vi "zatezovaci_charakteristika.vi"() -> ()   [LabVIEW 2024]
uses:
  <vilib>/Analysis/baseanly.llb/Mean (DBL).vi
  EFmeter.lvlib
  <vilib>/Analysis/NI_AALBase.lvlib
  BK Precision 8500B Series/BK Precision 8500B Series.lvlib
  <instrlib>/Zatez Kopper/Zatez Kopper.lvlib
panel:
  in  "LOAD":refnum<visa-resource-name>
  in  "Clear":bool
  in  "Typ zateze":u16(ring) items=["Manualni", "BK 8542B", "KOPPER-zatez"]
  in  "Ulozit data":bool caption="Uložit data"
  in  "file path (use dialog)":path
  in  "Vzorku na krokù":u16 max=100 step=1
  in  "Prumerovani":bool
  in  "Start [A]":dbl
  in  "Velikost kroku [A]":dbl
  in  "EFmeter":refnum<visa-resource-name>
  out "Aktualni zatez":dbl=2.5
  out "R_out":dbl
  in  "Pocet kroku":i32
  out "Zatezovaci charakteristika":cluster{"X":dbl[], "Y":dbl[]}[](graph)
  in  "stop":bool
  in  "Start":bool
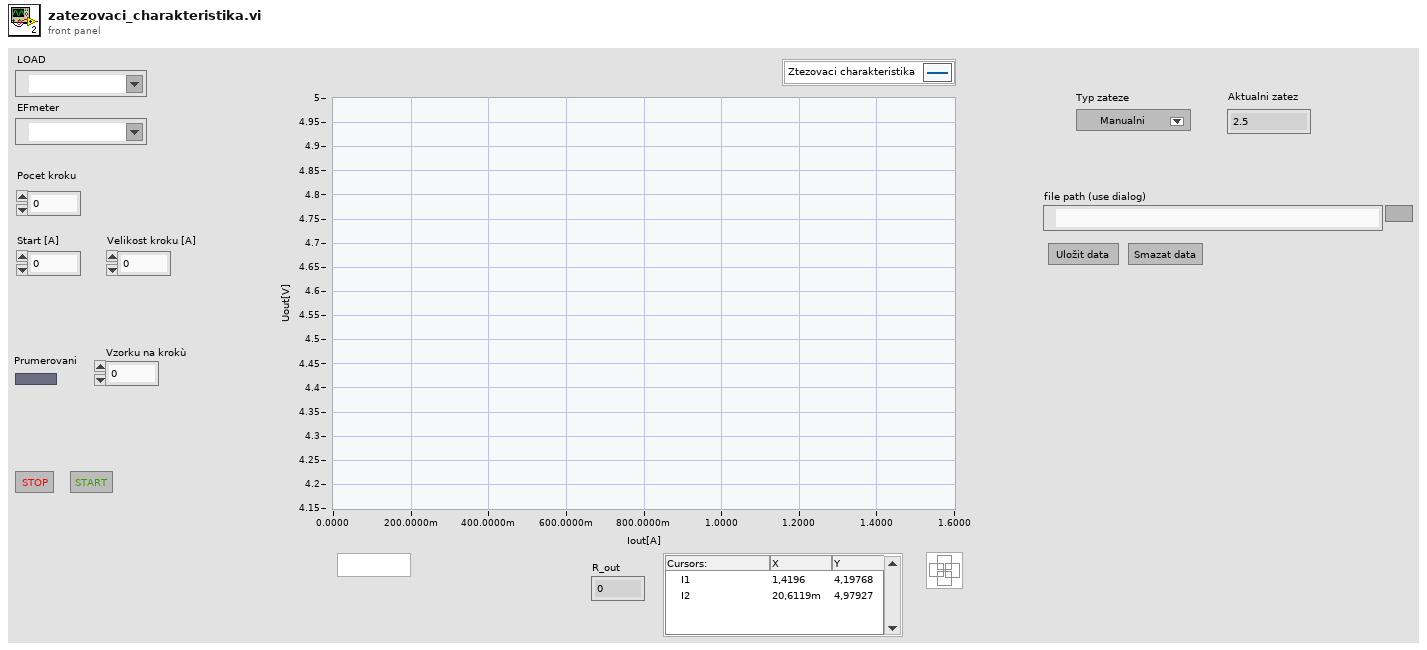
[diagram p1: front panel]
types:
  T1 = enum16{"init", "wait", "graph", "meas", "change_load", "init_measurment", "save", "clear"}
  T2 = typedef "LVCursorListTypeDef.ctl" = cluster{"Name":string, "Color":u32, "Style":u8, "Point Style":u8, "Name Visible":bool, "Allow Drag":bool, "Cursor Mode":u32, "Plot":i32, "Index":i32, "Position":cluster{"X":dbl, "Y":dbl}, "X Scale":u32, "Y Scale":u32, "Watch Plots":i32[], "Watch All Plots":bool, "Plot Area":i32, "Label Offset":cluster{"X":dbl, "Y":dbl}}[]
  T3 = cluster{"Name":string, "Color":u32, "Style":u8, "Point Style":u8, "Name Visible":bool, "Allow Drag":bool, "Cursor Mode":u32, "Plot":i32, "Index":i32, "Position":cluster{"X":dbl, "Y":dbl}, "X Scale":u32, "Y Scale":u32, "Watch Plots":i32[], "Watch All Plots":bool, "Plot Area":i32, "Label Offset":cluster{"X":dbl, "Y":dbl}}
  T4 = enum16{"open", "replace", "create", "open or create", "replace or create", "replace or create with confirmation"}
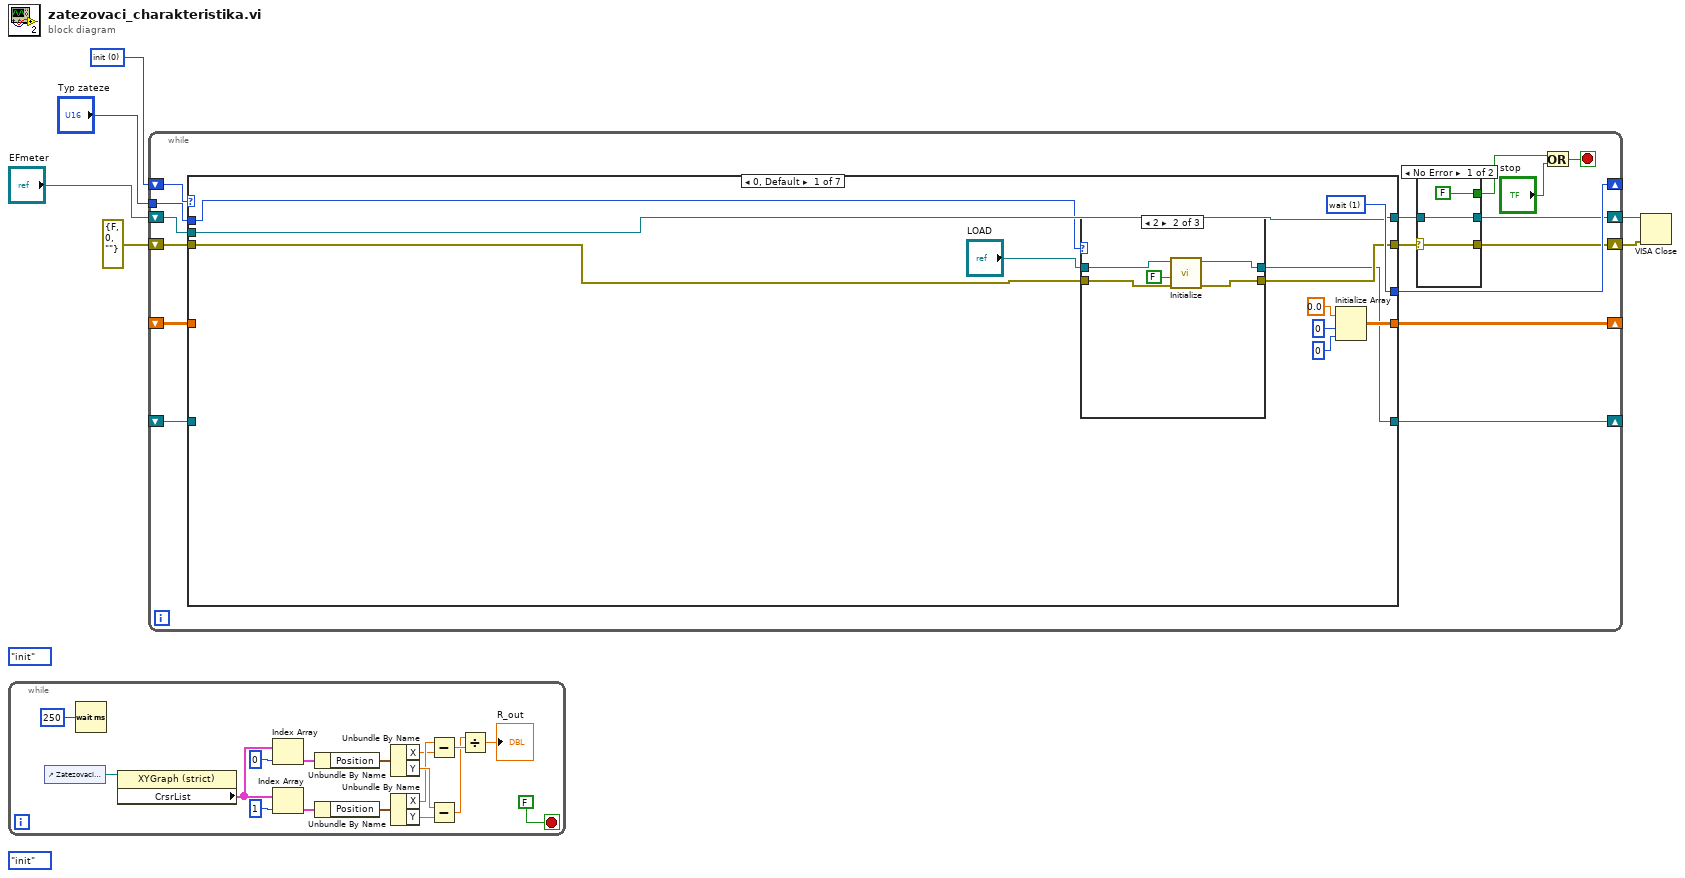
[diagram p0: block diagram]
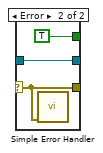
[diagram p2: hidden frame]
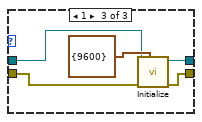
[diagram p4: hidden frame]
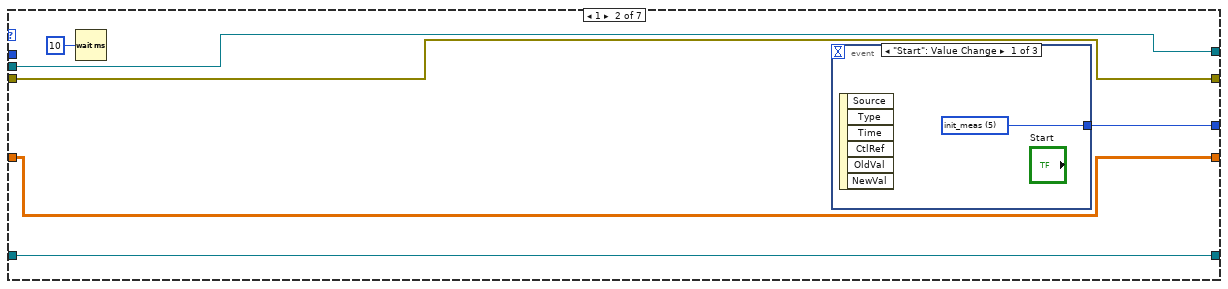
[diagram p5: hidden frame]
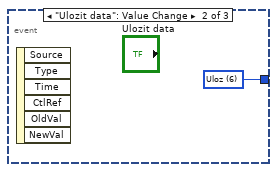
[diagram p6: hidden frame]
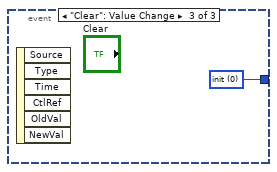
[diagram p7: hidden frame]
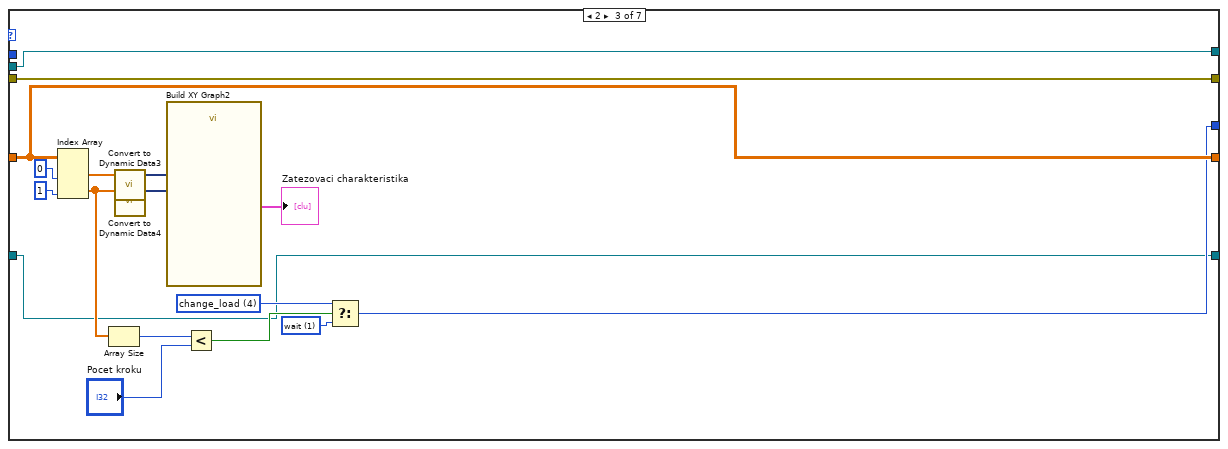
[diagram p8: hidden frame]
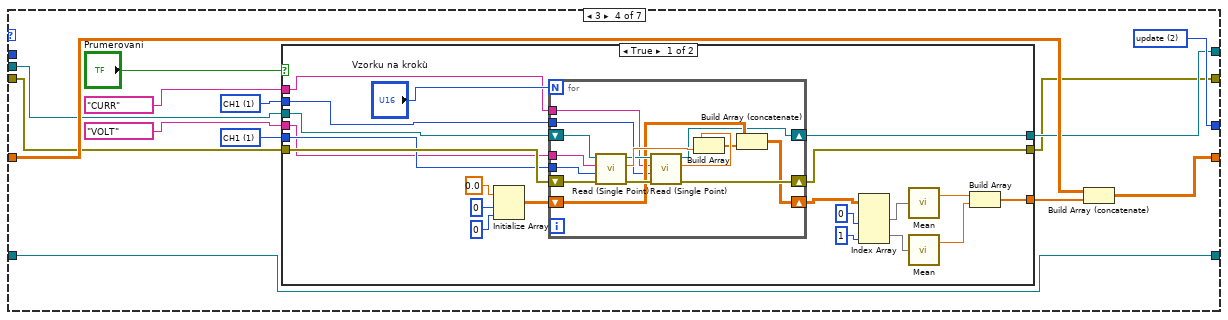
[diagram p9: hidden frame]
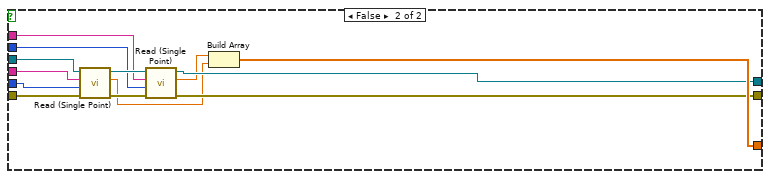
[diagram p10: hidden frame]
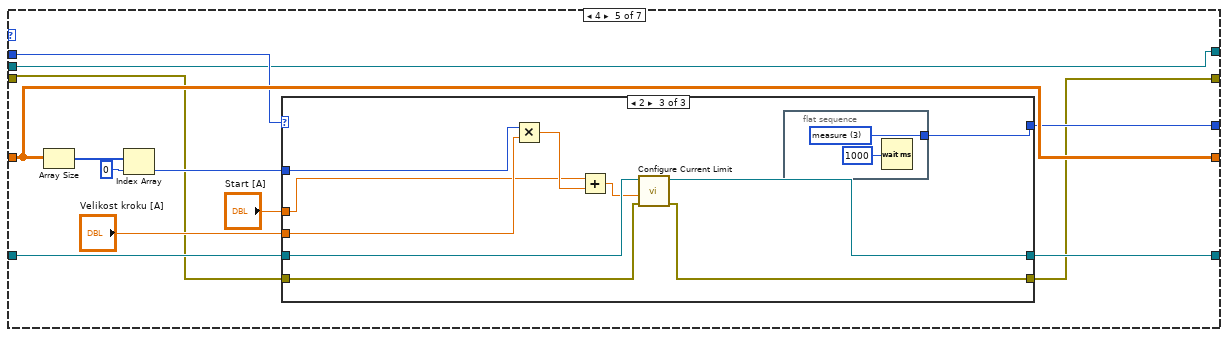
[diagram p11: hidden frame]
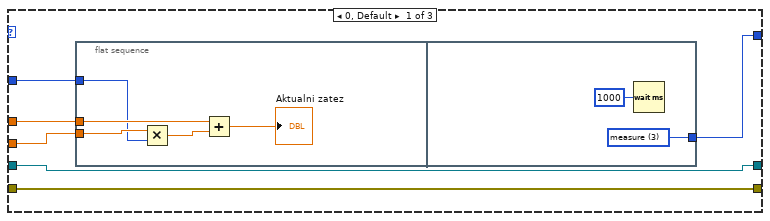
[diagram p12: hidden frame]
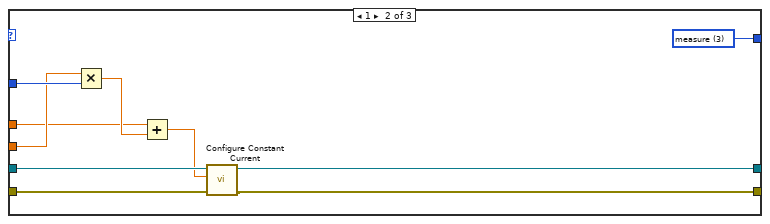
[diagram p13: hidden frame]
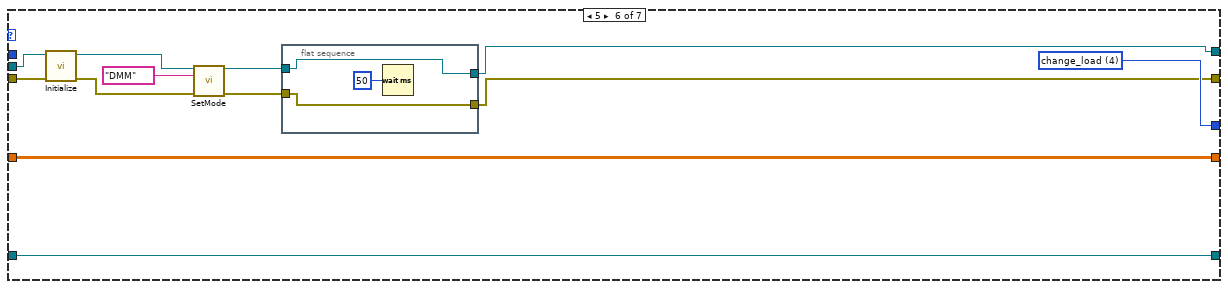
[diagram p14: hidden frame]
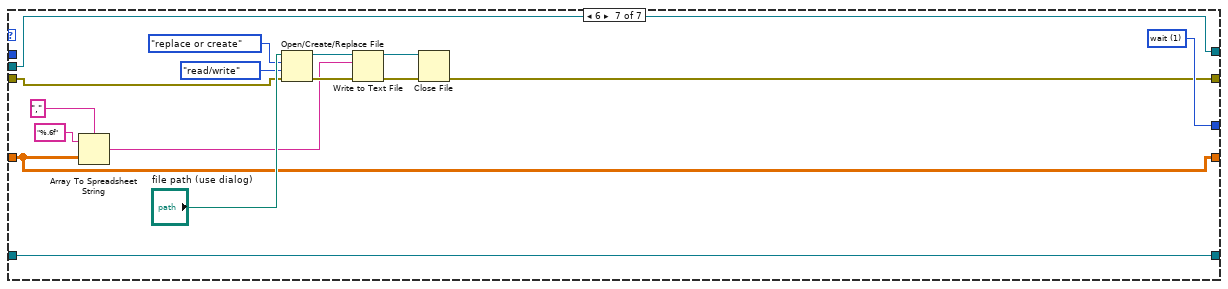
[diagram p15: hidden frame]
diagram:
  (unwired) T1."init"
  (unwired) T1."init"
  w6 = u16 0 items=["init", "wait", "update", "measure", "change_load", "init_meas", "Uloz", "clear"]
  n1 = while {
    stop <- FALSE stop-if-true
    n2 = control-ref of="Zatezovaci charakteristika"() -> (w21:refnum<vi>)
    n3 = Wait (ms)(milliseconds to wait=u32 250) -> ()  [unwired: 1 out]
    n4 = property class="XYGraph (strict)"(reference=w21) -> ("CrsrList"=w16:T2)  [unwired: 1 in, 2 out]
    n5 = Index Array(array=w16, index=0) -> (element=w22:T3)
    n6 = Index Array(array=w16, index=1) -> (element=w18:T3)
    n7 = Unbundle By Name(w22) -> ("Position"=w23:cluster{"X":dbl, "Y":dbl})
    n8 = Unbundle By Name(w18) -> ("Position"=w19:cluster{"X":dbl, "Y":dbl})
    n9 = Unbundle By Name(w23) -> ("X"=w7:dbl, "Y"=w14:dbl)
    n10 = Unbundle By Name(w19) -> ("X"=w8:dbl, "Y"=w15:dbl)
    n11 = Subtract(x=w8, y=w7) -> (x-y=w10:dbl)
    n12 = Subtract(x=w14, y=w15) -> (x-y=w9:dbl)
    n13 = Divide(x=w9, y=w10) -> (x/y=→"R_out":dbl)
  }
  n14 = while {
    shift-right: [w39] -> _
    shift-left: _ -> [w38]
    shift-right: [w34] -> _
    shift-left: w6 -> [w37]
    shift-right: [w31] -> w3
    shift-left: "EFmeter" -> [w36]
    shift-right: [w30] -> w2
    shift-left: errorcluster {"status"=FALSE, "code"=0, "source"=""} ("error in (no error)") -> [w35]
    tunnel: "Typ zateze" -> [w26]
    shift-right: [w25] -> _
    shift-left: _ -> [w24]
    stop <- w28 stop-if-true
    n15 = case shown="0, Default" w37 {
      tunnel: [w54 w73 w86 w107 w170 w217 w231] -> w39
      tunnel: w38 -> [_ w73 w86 w108 w170 w217 w231]
      tunnel: [w53 w74 w85 w105 w168 w211 w229] -> w34
      tunnel: [w49 w71 w79 w97 w158 w208 w225] -> w33
      tunnel: [w51 w72 w80 w98 w167 w210 w236] -> w32
      tunnel: w36 -> [w51 w72 w80 w104 w167 w213 w236]
      tunnel: w35 -> [w50 w71 w79 w103 w159 w212 w232]
      tunnel: w26 -> [w46 _ _ _ w169 _ _]
      tunnel: [w48 w69 w78 w95 w165 w206 w221] -> w25
      tunnel: w24 -> [_ w69 w78 w95 w166 w206 w221]
      frame 0, Default {
        w53 = u16 1 items=["init", "wait", "update", "measure"]
        n16 = case shown="2" w46 {
          tunnel: w50 -> [w58 w62 w67]
          tunnel: [w58 w61 w66] -> w49
          tunnel: [w57 w60 w65] -> w48
          tunnel: "LOAD" -> [w57 w63 w64]
          frame 0, Default {
          }
          frame 2 {
            n17 = call <instrlib>:"Initialize.vi"("error in (no error)"=w62, "Reset (True)"=FALSE, "VISA resource name"=w63) -> ("error out"=w61:errorcluster, "VISA resource name out"=w60:refnum<visa-resource-name>)  [unwired: 7 in]
          }
          frame 1 {
            n18 = call <instrlib>:"Initialize.vi"("Serial Configuration"=cluster{"Baud Rate":u32} {"Baud Rate"=9600}, "error in (no error)"=w67, "VISA resource name"=w64) -> ("error out"=w66:errorcluster, "VISA resource name out"=w65:refnum<visa-resource-name>)  [unwired: 7 in]
          }
        }
        n19 = Initialize Array(0.0 ("element"), 0 ("dimension size"), 0 ("dimension size")) -> (w54:dbl[][])
      }
      frame 1 {
        n20 = Wait (ms)(milliseconds to wait=u32 10) -> ()  [unwired: 1 out]
        n21 = event shown="[0] \"Start\": Value Change" {
          selector: _ -> [_ _ _]
          dyn-events: _ -> [_ _ _]
          timeout: _ -> [_ _ _]
          tunnel: [w75 w76 w77] -> w74
          event "Start": Value Change {
            w75 = u16 5 items=["init", "wait", "update", "measure", "change_load", "init_meas"]
            n22 = event-data() -> ()  [unwired: 1 in, 6 out]
          }
          event "Ulozit data": Value Change {
            w76 = u16 6 items=["init", "wait", "update", "measure", "change_load", "init_meas", "Uloz"]
            n23 = event-data() -> ()  [unwired: 1 in, 6 out]
          }
          event "Clear": Value Change {
            w77 = u16 0 items=["init", "wait", "update", "measure", "change_load", "init_meas", "Uloz", "clear"]
            n24 = event-data() -> ()  [unwired: 1 in, 6 out]
          }
        }
      }
      frame 2 {
        w81 = u16 4 items=["init", "wait", "update", "measure", "change_load", "init_meas"]
        w87 = u16 1 items=["init", "wait", "update", "measure"]
        n25 = Index Array(array=w86, index (col) #1=0 ("index (row)"), index (col) #2=1 ("index (row)")) -> (element #1=w94:dbl[], element #2=w89:dbl[])  [unwired: 2 in]
        n26 = Array Size(array=w89) -> (size(s)=w91:i32)
        n27 = call "Convert to Dynamic Data3"("Array"=w94) -> ("Dynamic Data Type"=w93:dynamicdata)  [unwired: 3 in]
        n28 = call "Convert to Dynamic Data4"("Array"=w89) -> ("Dynamic Data Type"=w92:dynamicdata)  [unwired: 3 in]
        n29 = call "Build XY Graph2"("Y Input"=w92, "X Input"=w93) -> ("XY Graph"=→"Zatezovaci charakteristika":cluster{"X":dbl[], "Y":dbl[]}[])  [unwired: 8 in, 1 out]
        n30 = Less?(x=w91, y="Pocet kroku") -> (x < y?=w90:bool)
        n31 = Select(t=w81, s=w90, f=w87) -> (s? t:f=w85:u16)
      }
      frame 3 {
        w99 = u16 1 items=["CH2"=2, "CH1"=1] ("Ring")
        w102 = u16 1 items=["CH2"=2, "CH1"=1] ("Ring")
        w105 = u16 2 items=["init", "wait", "update", "measure"]
        n32 = case shown="True" "Prumerovani" {
          tunnel: [w111 w157] -> w106
          tunnel: w104 -> [w124 w156]
          tunnel: w103 -> [w123 w155]
          tunnel: w102 -> [w122 w154]
          tunnel: "VOLT" ("Combo Box") -> [w121 w153]
          tunnel: "CURR" ("Combo Box") -> [w120 w150]
          tunnel: w99 -> [w119 w149]
          tunnel: [w110 w148] -> w98
          tunnel: [w109 w147] -> w97
          frame True {
            n33 = Initialize Array(0.0 ("element"), 0 ("dimension size"), 0 ("dimension size")) -> (w125:dbl[][])
            n34 = for {
              N: "Vzorku na krokù" -> [_]
              shift-right: [w137] -> w110
              shift-left: w124 -> [w138]
              shift-right: [w135] -> w109
              shift-left: w123 -> [w136]
              tunnel: w122 -> [w134]
              tunnel: w121 -> [w133]
              tunnel: w120 -> [w132]
              tunnel: w119 -> [w131]
              shift-right: [w130] -> w118
              shift-left: w125 -> [w139]
              n35 = call "Read (Single Point).vi"("error in (no error)"=w136, "Ring"=w134, "Combo Box"=w133, "VISA resource name"=w138) -> ("error out"=w142:errorcluster, "Measurement"=w144:dbl, "VISA resource name out"=w143:refnum<visa-resource-name>)  [unwired: 5 in]
              n36 = call "Read (Single Point).vi"("error in (no error)"=w142, "Ring"=w131, "Combo Box"=w132, "VISA resource name"=w143) -> ("error out"=w135:errorcluster, "Measurement"=w141:dbl, "VISA resource name out"=w137:refnum<visa-resource-name>)  [unwired: 5 in]
              n37 = Build Array(w141, w144) -> (w140:dbl[])
              n38 = Build Array (concatenate)(w139, w140) -> (w130:dbl[][])
            }
            n39 = Index Array(array=w118, index (col) #1=0 ("disabled index (col)"), index (col) #2=1 ("index (col)")) -> (element #1=w117:dbl[], element #2=w116:dbl[])  [unwired: 2 in]
            n40 = call-poly <vilib>:"Mean.vi"("X"=w117) -> ("mean"=w113:dbl)  [unwired: 1 out]
            n41 = call-poly <vilib>:"Mean.vi"("X"=w116) -> ("mean"=w112:dbl)  [unwired: 1 out]
            n42 = Build Array(w113, w112) -> (w111:dbl[])
          }
          frame False {
            n43 = call "Read (Single Point).vi"("error in (no error)"=w155, "Ring"=w154, "Combo Box"=w153, "VISA resource name"=w156) -> ("error out"=w152:errorcluster, "Measurement"=w145:dbl, "VISA resource name out"=w151:refnum<visa-resource-name>)  [unwired: 5 in]
            n44 = call "Read (Single Point).vi"("error in (no error)"=w152, "Ring"=w149, "Combo Box"=w150, "VISA resource name"=w151) -> ("error out"=w147:errorcluster, "Measurement"=w146:dbl, "VISA resource name out"=w148:refnum<visa-resource-name>)  [unwired: 5 in]
            n45 = Build Array(w146, w145) -> (w157:dbl[])
          }
        }
        n46 = Build Array (concatenate)(w108, w106) -> (w107:dbl[][])
      }
      frame 4 {
        n47 = Array Size(array=w170) -> (size(s)=w160:i32[])
        n48 = Index Array(array=w160, index=0) -> (element=w162:i32)
        n49 = case shown="2" w169 {
          tunnel: [w176 w193 w194] -> w168
          tunnel: w166 -> [w175 w192 w200]
          tunnel: [w175 w191 w203] -> w165
          tunnel: "Velikost kroku [A]" -> [w174 w189 w198]
          tunnel: "Start [A]" -> [w173 w187 w197]
          tunnel: w162 -> [w172 w190 w195]
          tunnel: w159 -> [w171 w185 w201]
          tunnel: [w171 w184 w202] -> w158
          frame 0, Default {
            n50 = flat-sequence {
              tunnel: w174 -> [w179]
              tunnel: w173 -> [w178]
              tunnel: w172 -> [w177]
              tunnel: [w183] -> w176
              frame #0 {
                n51 = Multiply(x=w179, y=w177) -> (x*y=w181:dbl)
                n52 = Add(x=w178, y=w181) -> (x+y=→"Aktualni zatez":dbl)
              }
              frame #1 {
                w183 = u16 3 items=["init", "wait", "update", "measure", "change_load", "init_meas"]
                n53 = Wait (ms)(milliseconds to wait=u32 1000) -> ()  [unwired: 1 out]
              }
            }
          }
          frame 1 {
            w193 = u16 3 items=["init", "wait", "update", "measure", "change_load", "init_meas"]
            n54 = Multiply(x=w189, y=w190) -> (x*y=w188:dbl)
            n55 = Add(x=w187, y=w188) -> (x+y=w186:dbl)
            n56 = call "Configure Constant Current.vi"("error in (no error)"=w185, "CC Current (0)"=w186, "VISA resource name"=w192) -> ("error out"=w184:errorcluster, "VISA resource name out"=w191:refnum<visa-resource-name>)  [unwired: 7 in]
          }
          frame 2 {
            n57 = Multiply(x=w195, y=w198) -> (x*y=w199:dbl)
            n58 = Add(x=w197, y=w199) -> (x+y=w196:dbl)
            n59 = call <instrlib>:"Configure Current Limit.vi"("error in (no error)"=w201, "Current Limit (0.0 A)"=w196, "VISA resource name"=w200) -> ("error out"=w202:errorcluster, "VISA resource name out"=w203:refnum<visa-resource-name>)  [unwired: 7 in]
            n60 = flat-sequence {
              tunnel: [w205] -> w194
              frame #0 {
                w205 = u16 3 items=["init", "wait", "update", "measure", "change_load", "init_meas"]
                n61 = Wait (ms)(milliseconds to wait=u32 1000) -> ()  [unwired: 1 out]
              }
            }
          }
        }
      }
      frame 5 {
        w211 = u16 4 items=["init", "wait", "update", "measure", "change_load", "init_meas"]
        n62 = call <instrlib>:"Initialize.vi"("error in (no error)"=w212, "VISA resource name"=w213) -> ("error out"=w216:errorcluster, "VISA resource name out"=w215:refnum<visa-resource-name>)  [unwired: 8 in]
        n63 = call "SetMode.vi"("VISA resource name"=w215, "Combo Box"="DMM", "error in (no error)"=w216) -> ("VISA resource name out"=w209:refnum<visa-resource-name>, "error out"=w207:errorcluster)  [unwired: 11 in]
        n64 = flat-sequence {
          tunnel: [w219] -> w210
          tunnel: w209 -> [w219]
          tunnel: w207 -> [w218]
          tunnel: [w218] -> w208
          frame #0 {
            n65 = Wait (ms)(milliseconds to wait=u32 50) -> ()  [unwired: 1 out]
          }
        }
      }
      frame 6 {
        w229 = u16 1 items=["init", "wait", "update", "measure", "change_load", "init_meas"]
        n66 = Array To Spreadsheet String(delimiter (Tab)=",", array=w231, 3:"%.6f" ("format string")) -> (spreadsheet string=w222:string)
        n67 = Open/Create/Replace File(file path (use dialog)="file path (use dialog)", error in=w232, operation (0:open)=T4."replace or create", access (0:read/write)=enum16{"read/write", "read-only", "write-only"}."read/write") -> (refnum out=w224:refnum<file>, error out=w227:errorcluster)  [unwired: 2 in, 1 out]
        n68 = Write to Text File(file (use dialog)=w224, text=w222, error in=w227) -> (refnum out=w223:refnum<file>, error out=w226:errorcluster)  [unwired: 1 in, 1 out]
        n69 = Close File(refnum=w223, error in=w226) -> (error out=w225:errorcluster)  [unwired: 1 out]
      }
    }
    n70 = case shown="No Error" w33 {
      selector: w33 -> [w41 w43]
      tunnel: w32 -> [w42 w45]
      tunnel: [w42 w45] -> w31
      tunnel: [w41 w43] -> w30
      tunnel: [FALSE TRUE] -> w27
      frame No Error {
      }
      frame Error {
        n71 = call <vilib>:"Simple Error Handler.vi"("error in (no error)"=w43) -> ()  [unwired: 4 in, 5 out]
      }
    }
    n72 = Or(x=w27, y="stop") -> (x .or. y?=w28:bool)
  }
  n73 = VISA Close(VISA resource name=w3, error in (no error)=w2) -> ()  [unwired: 1 out]
